vi "Msg To Self.vi"(9 "Priority?":bool, 10 "Msg":refnum<class "Msg.lvclass">, 11 "Dev Panel in":refnum<class "Dev Panel.lvclass">) -> (0 "error out":errorcluster)   [LabVIEW 2021, in "Dev Panel.lvclass"]
uses:
  Dev Panel.lvclass
  Dev Panel.lvclass/Dev Panel.ctl
  Actor/Actor/Actor.lvclass
  Actor/Msg/Msg.lvclass
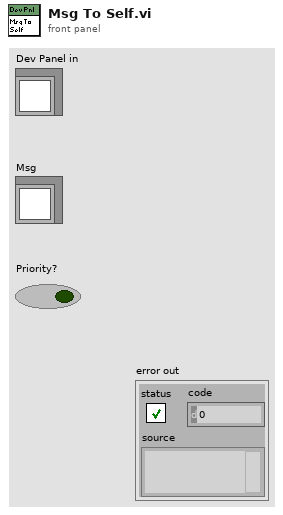
[diagram p1: front panel]
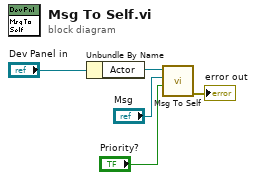
[diagram p0: block diagram]
diagram:
  n1 = Unbundle By Name("Dev Panel in") -> ("Actor"=w4:refnum<class "Actor.lvclass">)
  n2 = call-dynamic "Msg To Self.vi"("Priority?"="Priority?", "Msg"="Msg", "Actor in"=w4) -> ("error out"=→"error out":errorcluster)  [unwired: 8 in]
